vi "Подзавод.vi"(10 "Хранилище in":T1, 11 "Количество":dbl) -> (3 "Хранилище out":T1)   [LabVIEW 2021]
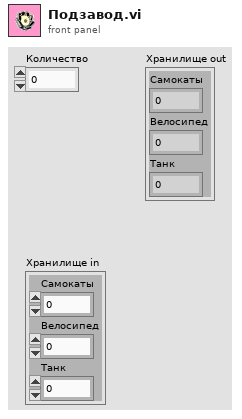
[diagram p1: front panel]
types:
  T1 = cluster{"Самокаты":dbl, "Велосипед":dbl, "Танк":dbl}
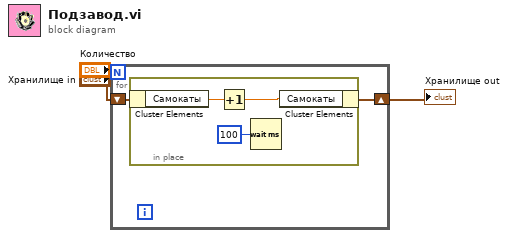
[diagram p0: block diagram]
diagram:
  n1 = for {
    N: "Количество" -> [_]
    shift-right: [w4] -> w3
    shift-left: "Хранилище in" -> [w5]
    n2 = in-place {
      n3 = in-place-cluster #1(w5) -> ("Самокаты"=w8:dbl)
      n4 = Increment(x=w8) -> (x+1=w7:dbl)
      n5 = Wait (ms)(milliseconds to wait=u32 100) -> ()  [unwired: 1 out]
      n6 = in-place-cluster #1("Самокаты"=w7) -> (w4:T1)
    }
  }
  "Хранилище out" <- w3
